vi "LoadArmPressureWrapper.vi"(8 "error in":errorcluster, 11 "File dir":path) -> (0 "error out":errorcluster, 2 "Armpressure Left":T1(array[cluster]), 3 "Armpressure Right":T1(array[cluster]))   [LabVIEW 2013, in "main.lvlib"]
uses:
  main.lvlib
  <userlib>/_OpenG.lib/file/file.llb/File Exists - Scalar__ogtk.vi
  Globals/DataPathGlobalVariable.vi
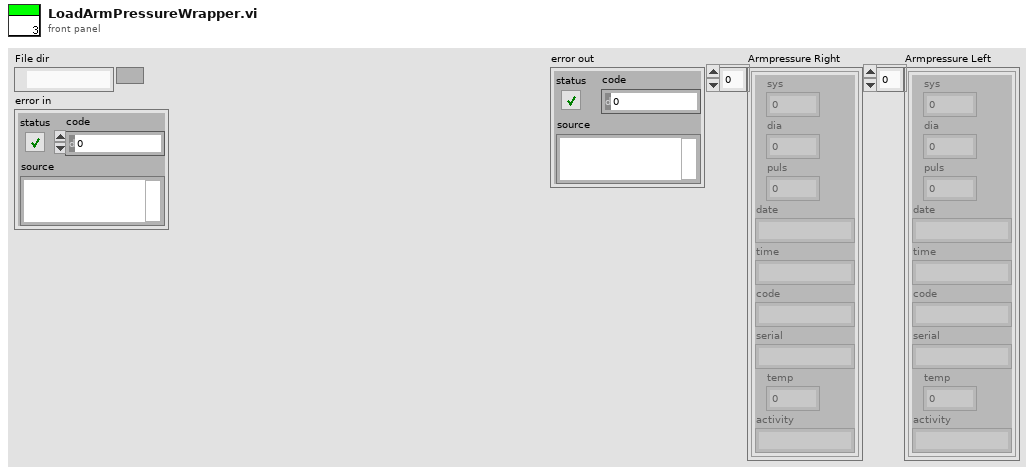
[diagram p1: front panel]
types:
  T1 = cluster{"sys":dbl, "dia":dbl, "puls":dbl, "date":string, "time":string, "code":string, "serial":string, "temp":dbl, "activity":string}[]
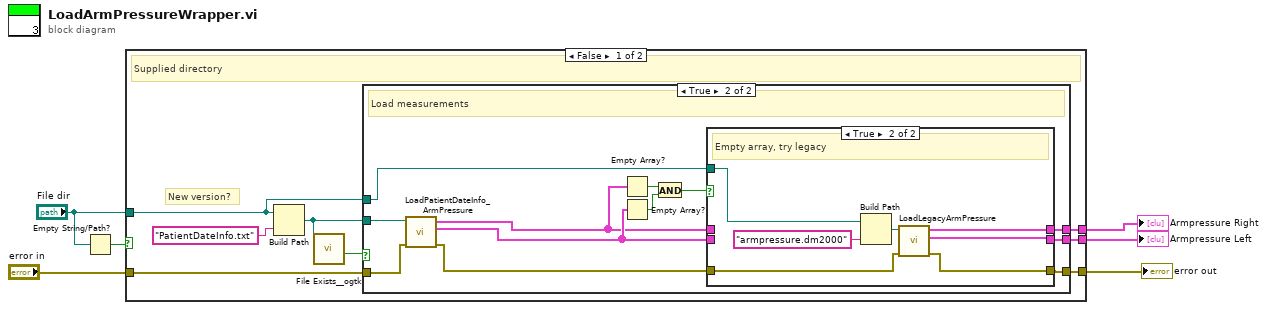
[diagram p0: block diagram]
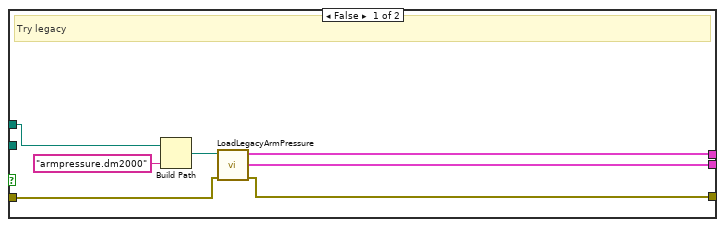
[diagram p2: hidden frame]
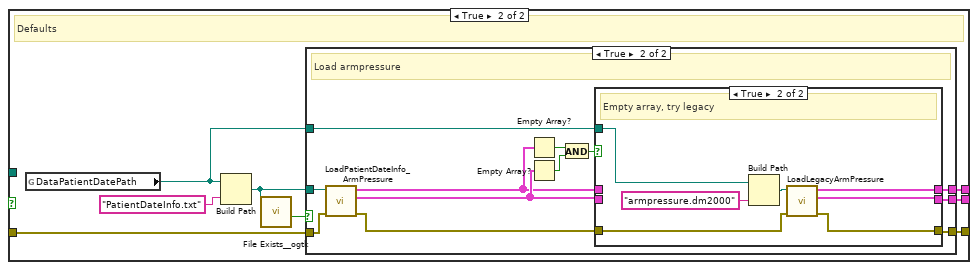
[diagram p4: hidden frame]
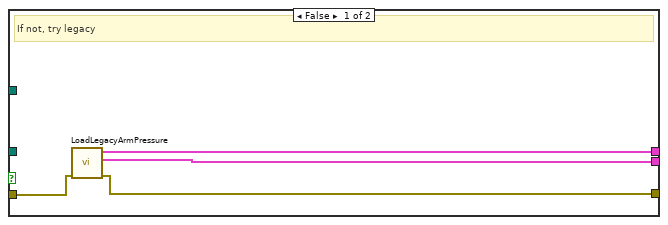
[diagram p5: hidden frame]
diagram:
  n1 = Empty String/Path?(string/path="File dir") -> (empty?=w6:bool)
  n2 = case shown="False" w6 {
    tunnel: [w11 w48] -> w5
    tunnel: [w10 w47] -> w4
    tunnel: "File dir" -> [w7 _]
    tunnel: "error in" -> [w9 w46]
    tunnel: [w8 w45] -> w1
    frame False {
      # "New version?"
      # "Supplied directory"
      n3 = Build Path(base path=w7, name or relative path="PatientDateInfo.txt") -> (appended path=w12:path)
      n4 = call-poly <userlib>:"File Exists__ogtk.vi"("file path"=w12) -> ("exists"=w13:bool)  [unwired: 6 in, 1 out]
      n5 = case shown="True" w13 {
        tunnel: w12 -> [_ w33]
        tunnel: [w19 w25] -> w11
        tunnel: [w18 w26] -> w10
        tunnel: w9 -> [w17 w32]
        tunnel: [w16 w22] -> w8
        tunnel: w7 -> [w15 w28]
        frame False {
          # "Try legacy"
          n6 = Build Path(base path=w15, name or relative path="armpressure.dm2000") -> (appended path=w20:path)
          n7 = call "LoadLegacyArmPressure.vi"("error in (no error)"=w17, "File path"=w20) -> ("error out"=w16:errorcluster, "Left"=w18:T1, "Right"=w19:T1)  [unwired: 7 in]
        }
        frame True {
          # "Load measurements"
          n8 = call "LoadPatientDateInfo_ArmPressure.vi"("error in"=w32, "File path"=w33) -> ("error out"=w23:errorcluster, "Armpressure Left"=w27:T1, "Armpressure Right"=w24:T1)  [unwired: 7 in]
          n9 = Empty Array?(array=w24) -> (empty?=w30:bool)
          n10 = Empty Array?(array=w27) -> (empty?=w31:bool)
          n11 = And(x=w30, y=w31) -> (x .and. y?=w29:bool)
          n12 = case shown="True" w29 {
            tunnel: w28 -> [_ w41]
            tunnel: w27 -> [w36 _]
            tunnel: [w36 w39] -> w26
            tunnel: [w35 w40] -> w25
            tunnel: w24 -> [w35 _]
            tunnel: [w34 w38] -> w22
            tunnel: w23 -> [w34 w37]
            frame False {
            }
            frame True {
              # "Empty array, try legacy"
              n13 = Build Path(base path=w41, name or relative path="armpressure.dm2000") -> (appended path=w42:path)
              n14 = call "LoadLegacyArmPressure.vi"("error in (no error)"=w37, "File path"=w42) -> ("error out"=w38:errorcluster, "Left"=w39:T1, "Right"=w40:T1)  [unwired: 7 in]
            }
          }
        }
      }
    }
    frame True {
      # "Defaults"
      n15 = global read "DataPathGlobalVariable.vi" "DataPatientDatePath"() -> (w44:path)
      n16 = Build Path(base path=w44, name or relative path="PatientDateInfo.txt") -> (appended path=w49:path)
      n17 = call-poly <userlib>:"File Exists__ogtk.vi"("file path"=w49) -> ("exists"=w50:bool)  [unwired: 6 in, 1 out]
      n18 = case shown="True" w50 {
        tunnel: w49 -> [_ w67]
        tunnel: [w55 w64] -> w48
        tunnel: [w54 w63] -> w47
        tunnel: w46 -> [w53 w66]
        tunnel: [w52 w62] -> w45
        tunnel: w44 -> [_ w65]
        frame False {
          # "If not, try legacy"
          n19 = call "LoadLegacyArmPressure.vi"("error in (no error)"=w53) -> ("error out"=w52:errorcluster, "Left"=w54:T1, "Right"=w55:T1)  [unwired: 8 in]
        }
        frame True {
          # "Load armpressure"
          n20 = call "LoadPatientDateInfo_ArmPressure.vi"("error in"=w66, "File path"=w67) -> ("error out"=w61:errorcluster, "Armpressure Left"=w57:T1, "Armpressure Right"=w56:T1)  [unwired: 7 in]
          n21 = Empty Array?(array=w56) -> (empty?=w59:bool)
          n22 = Empty Array?(array=w57) -> (empty?=w60:bool)
          n23 = And(x=w59, y=w60) -> (x .and. y?=w58:bool)
          n24 = case shown="True" w58 {
            tunnel: w65 -> [_ w75]
            tunnel: w57 -> [w70 _]
            tunnel: [w70 w73] -> w63
            tunnel: [w69 w74] -> w64
            tunnel: w56 -> [w69 _]
            tunnel: [w68 w72] -> w62
            tunnel: w61 -> [w68 w71]
            frame False {
            }
            frame True {
              # "Empty array, try legacy"
              n25 = Build Path(base path=w75, name or relative path="armpressure.dm2000") -> (appended path=w76:path)
              n26 = call "LoadLegacyArmPressure.vi"("error in (no error)"=w71, "File path"=w76) -> ("error out"=w72:errorcluster, "Left"=w73:T1, "Right"=w74:T1)  [unwired: 7 in]
            }
          }
        }
      }
    }
  }
  "error out" <- w1
  "Armpressure Right" <- w5
  "Armpressure Left" <- w4
